vi "equipment_2.vi"() -> ()   [LabVIEW 2016]
uses:
  <vilib>/Platform/TimedLoop/XDataNode/timing_clust.ctl
  <vilib>/Platform/TimedLoop/XDataNode/nitl_modes.ctl
  <vilib>/Platform/TimedLoop/XDataNode/wakeup.ctl
  <instrlib>/Lake Shore 425/Public/Data/Field Data (Single Reading).vi
  <vilib>/platform/TimedLoop/XDataNode/XDataNode.xnode
  <instrlib>/Lake Shore 425/Lake Shore 425.lvlib
  <vilib>/Platform/TimedLoop/XDataNode/XDNodeRunTimeDep.lvlib
panel:
  out "Array":T1(array[cluster])
  out "XY Graph":T1(graph)
  in  "Period (ms)":i64
  out "Error":errorcluster
  in  "stop":bool
  out "Waveform Chart":dbl(graph)
  out "error out 3":errorcluster
  out "error out 2":errorcluster
  out "error out 1":errorcluster
  out "Probe Sensitivity 3":dbl=0.001 format="%^.3e"
  out "Probe Serial Number 3":string
  out "Probe Type  3":u16(ring)=40 items=["High Sensitivity"=40, "High Stability"=41, "Ultra-High Sensitivity"=42, "User Programmable Cable / High Sensitivity Probe"=50, "User Programmable Cable / High Stability Probe"=51, "User Programmable Cable / Ultra-High Sensitivity Probe"=52]
  out "Probe Sensitivity 2":dbl=0.001 format="%^.3e"
  out "Probe Serial Number 2":string
  out "Probe Type  2":u16(ring)=40 items=["High Sensitivity"=40, "High Stability"=41, "Ultra-High Sensitivity"=42, "User Programmable Cable / High Sensitivity Probe"=50, "User Programmable Cable / High Stability Probe"=51, "User Programmable Cable / Ultra-High Sensitivity Probe"=52]
  out "Probe Sensitivity":dbl=0.001 format="%^.3e"
  out "Probe Serial Number":string
  out "Probe Type":u16(ring)=40 items=["High Sensitivity"=40, "High Stability"=41, "Ultra-High Sensitivity"=42, "User Programmable Cable / High Sensitivity Probe"=50, "User Programmable Cable / High Stability Probe"=51, "User Programmable Cable / Ultra-High Sensitivity Probe"=52]
  in  "VISA Gaussmeter 3":refnum<visa-resource-name>
  in  "VISA Gaussmeter 2":refnum<visa-resource-name>
  in  "VISA Gaussmeter 1":refnum<visa-resource-name>
  in  "Gaussmeter 3":bool
  in  "Gaussmeter 2":bool
  in  "Gaussmeter 1":bool
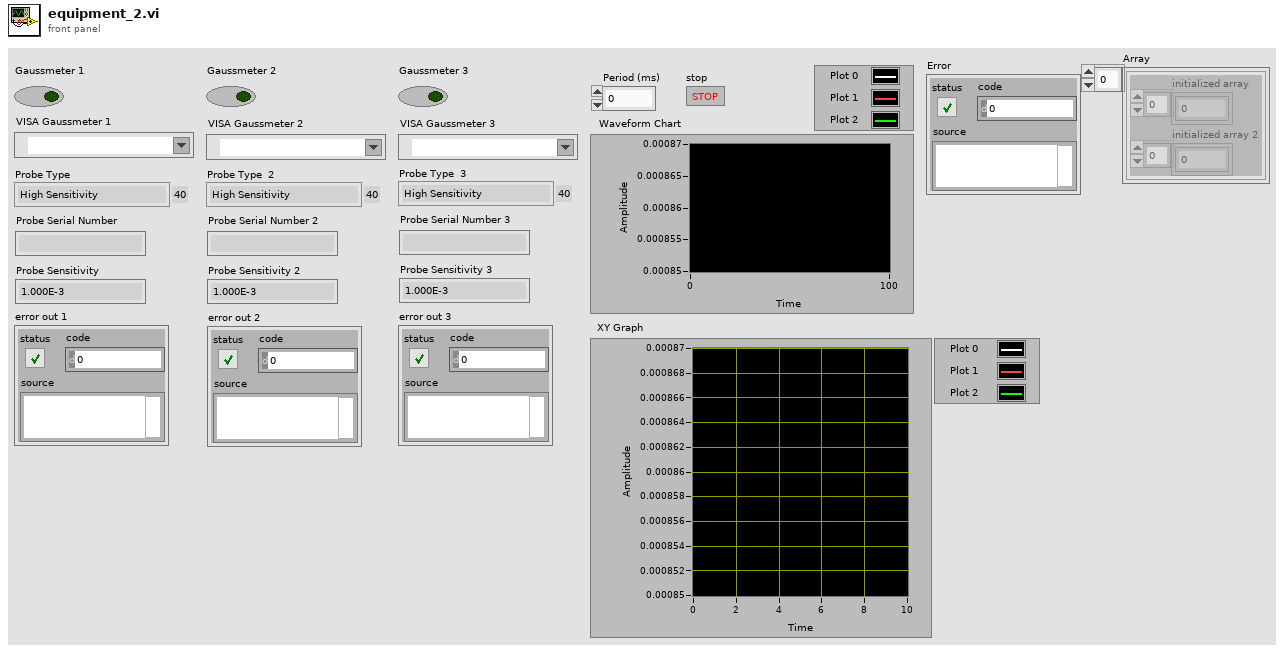
[diagram p1: front panel]
types:
  T1 = cluster{"initialized array":dbl[], "initialized array 2":dbl[]}[]
  T2 = typedef "XDNodeRunTimeDep.lvlib/timing_clust.ctl" = cluster{"Expected End [f-1]":u64, "Actual End [f-1]":u64, "Finished Late? [f-1]":bool, "Expected End [i-1]":u64, "Actual End [i-1]":u64, "Finished Late? [i-1]":bool, "Expected Start [i]":u64, "Actual Start [i]":u64, "Expected Start [f]":u64, "Actual Start [f]":u64, "Source Name":string, "Structure Name":string, "Period":i64, "Deadline":i64, "Offset":i64, "Start":i64, "Priority":i32, "Timeout":i32, "Mode":T3, "Wakeup Reason":T4, "Error":errorcluster, "Source Type":string, "Secondary Source Type":string, "Global End Time":u64, "Global Start Time":u64, "Frame Duration":u64, "Iteration Duration":u64, "Assigned CPU":i32, "I/O Scan Engine Mode":u32}
  T3 = typedef "XDNodeRunTimeDep.lvlib/nitl_modes.ctl" = enum32{"No Change", "Process missed periods, maintain original phase", "Discard missed periods, maintain original phase", "Process missed periods, ignore original phase", "Discard missed periods, ignore original phase"}
  T4 = typedef "XDNodeRunTimeDep.lvlib/wakeup.ctl" = enum32{"Normal", "Aborted", "Asynchronous wakeup", "Timing source error", "Timed loop error", "Timeout"}
  T5 = cluster{"initialized array":dbl[], "initialized array 2":dbl[]}
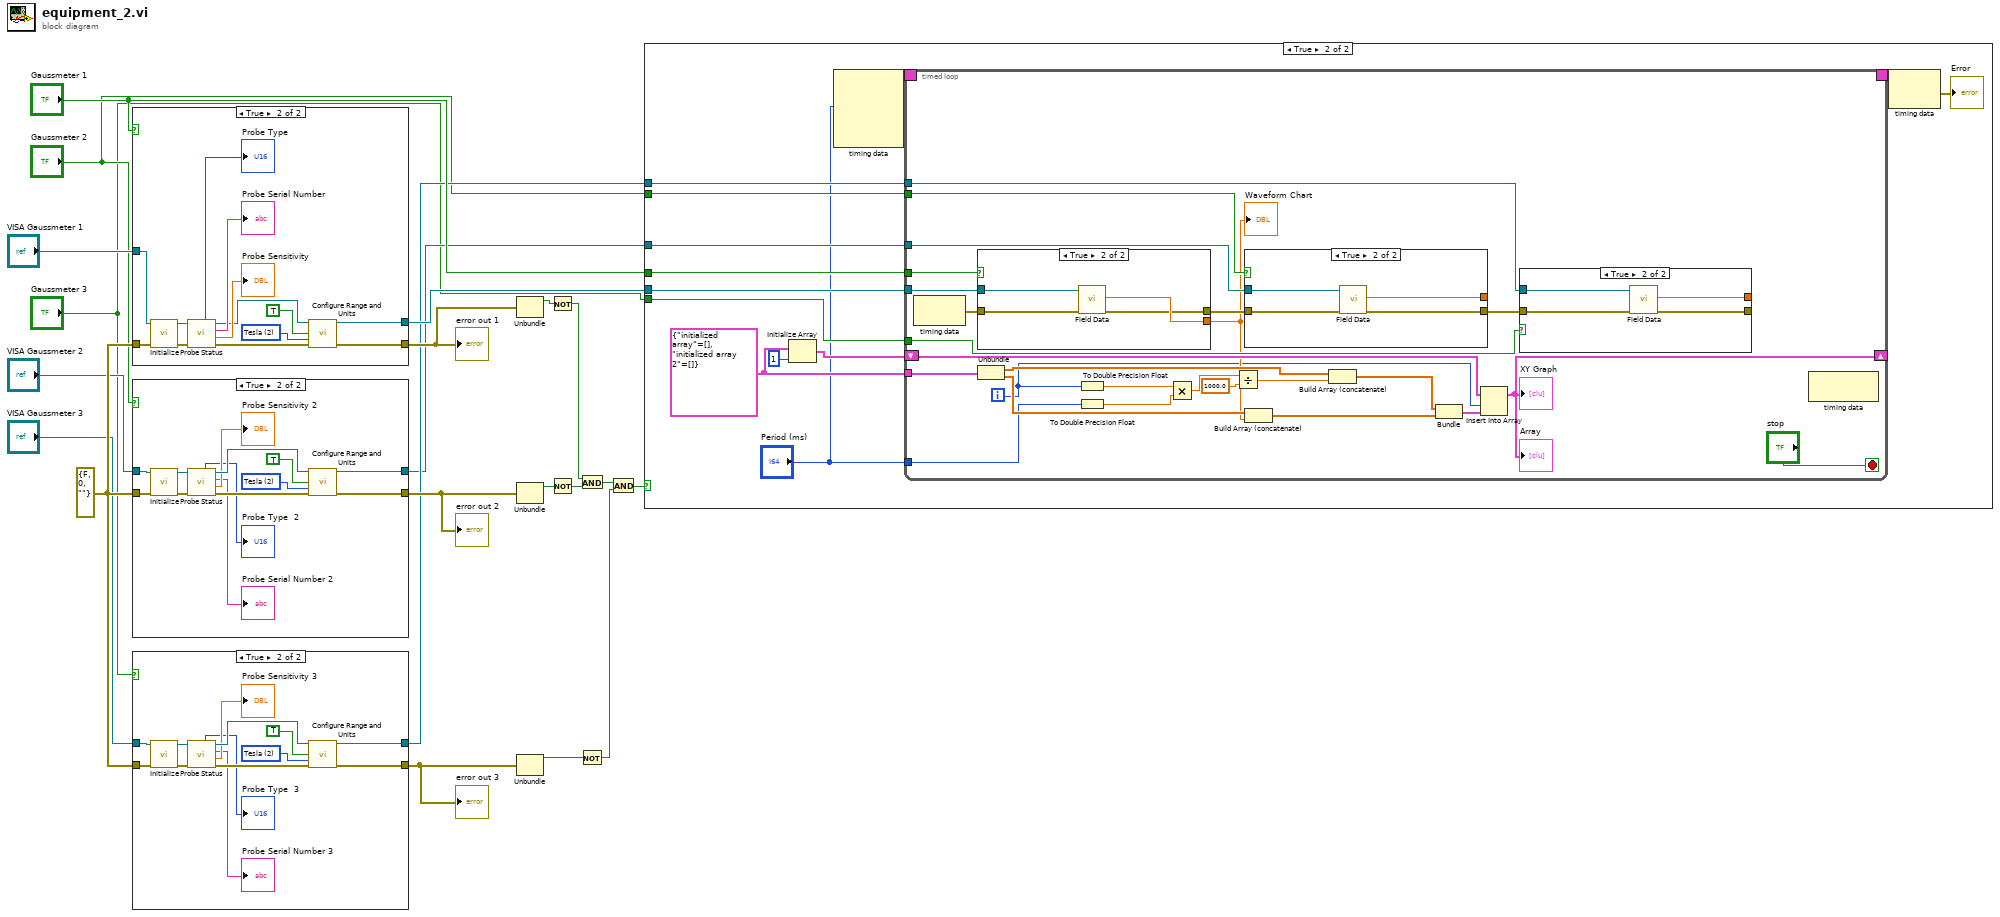
[diagram p0: block diagram]
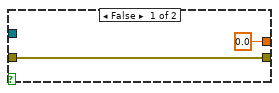
[diagram p3: hidden frame]
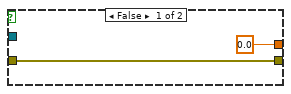
[diagram p4: hidden frame]
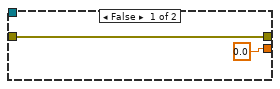
[diagram p5: hidden frame]
diagram:
  w21 = errorcluster {"status"=FALSE, "code"=0, "source"=""} ("error out")
  n1 = case shown="True" "Gaussmeter 1" {
    tunnel: [w23 w28] -> w15
    tunnel: w21 -> [w23 w36]
    tunnel: [w22 w25] -> w19
    tunnel: "VISA Gaussmeter 1" -> [w22 w24]
    frame False {
    }
    frame True {
      w26 = u16 2 items=["Gauss"=1, "Tesla"=2, "Oersted"=3, "Amp/meter"=4] ("Field Units (1:Gauss)")
      n2 = call <instrlib>:"Initialize.vi"("error in (no error)"=w36, "VISA resource name"=w24) -> ("error out"=w34:errorcluster, "VISA resource name out"=w35:refnum<visa-resource-name>)  [unwired: 8 in]
      n3 = call <instrlib>:"Probe Status.vi"("error in (no error)"=w34, "VISA resource name"=w35) -> ("error out"=w29:errorcluster, "Probe Sensitivity"=→"Probe Sensitivity":dbl, "Probe Serial Number"=→"Probe Serial Number":string, "VISA resource name out"=w30:refnum<visa-resource-name>, "Probe Type"=→"Probe Type":u16)  [unwired: 4 in, 1 out]
      n4 = call <instrlib>:"Configure Range and Units.vi"("VISA resource name"=w30, "Auto Range (F: Off)"=TRUE, "Field Units (1:Gauss)"=w26, "error in (no error)"=w29) -> ("VISA resource name out"=w25:refnum<visa-resource-name>, "error out"=w28:errorcluster)  [unwired: 10 in]
    }
  }
  "error out 1" <- w15
  n5 = case shown="True" "Gaussmeter 2" {
    tunnel: w21 -> [w38 w51]
    tunnel: [w38 w41] -> w14
    tunnel: "VISA Gaussmeter 2" -> [w37 w40]
    tunnel: [w37 w39] -> w3
    frame False {
    }
    frame True {
      w50 = u16 2 items=["Gauss"=1, "Tesla"=2, "Oersted"=3, "Amp/meter"=4] ("Field Units (1:Gauss)")
      n6 = call <instrlib>:"Initialize.vi"("error in (no error)"=w51, "VISA resource name"=w40) -> ("error out"=w42:errorcluster, "VISA resource name out"=w43:refnum<visa-resource-name>)  [unwired: 8 in]
      n7 = call <instrlib>:"Probe Status.vi"("error in (no error)"=w42, "VISA resource name"=w43) -> ("error out"=w48:errorcluster, "Probe Sensitivity"=→"Probe Sensitivity 2":dbl, "Probe Serial Number"=→"Probe Serial Number 2":string, "VISA resource name out"=w47:refnum<visa-resource-name>, "Probe Type"=→"Probe Type  2":u16)  [unwired: 4 in, 1 out]
      n8 = call <instrlib>:"Configure Range and Units.vi"("VISA resource name"=w47, "Auto Range (F: Off)"=TRUE, "Field Units (1:Gauss)"=w50, "error in (no error)"=w48) -> ("VISA resource name out"=w39:refnum<visa-resource-name>, "error out"=w41:errorcluster)  [unwired: 10 in]
    }
  }
  "error out 2" <- w14
  n9 = case shown="True" "Gaussmeter 3" {
    tunnel: w21 -> [w53 w66]
    tunnel: [w53 w58] -> w13
    tunnel: "VISA Gaussmeter 3" -> [w52 w55]
    tunnel: [w52 w54] -> w4
    frame False {
    }
    frame True {
      w65 = u16 2 items=["Gauss"=1, "Tesla"=2, "Oersted"=3, "Amp/meter"=4] ("Field Units (1:Gauss)")
      n10 = call <instrlib>:"Initialize.vi"("error in (no error)"=w66, "VISA resource name"=w55) -> ("error out"=w57:errorcluster, "VISA resource name out"=w56:refnum<visa-resource-name>)  [unwired: 8 in]
      n11 = call <instrlib>:"Probe Status.vi"("error in (no error)"=w57, "VISA resource name"=w56) -> ("error out"=w63:errorcluster, "Probe Sensitivity"=→"Probe Sensitivity 3":dbl, "Probe Serial Number"=→"Probe Serial Number 3":string, "VISA resource name out"=w62:refnum<visa-resource-name>, "Probe Type"=→"Probe Type  3":u16)  [unwired: 4 in, 1 out]
      n12 = call <instrlib>:"Configure Range and Units.vi"("VISA resource name"=w62, "Auto Range (F: Off)"=TRUE, "Field Units (1:Gauss)"=w65, "error in (no error)"=w63) -> ("VISA resource name out"=w54:refnum<visa-resource-name>, "error out"=w58:errorcluster)  [unwired: 10 in]
    }
  }
  "error out 3" <- w13
  n13 = Unbundle(w15) -> ("status"=w10:bool)  [unwired: 2 out]
  n14 = Unbundle(w14) -> ("status"=w8:bool)  [unwired: 2 out]
  n15 = Unbundle(w13) -> ("status"=w6:bool)  [unwired: 2 out]
  n16 = Not(x=w10) -> (.not. x?=w9:bool)
  n17 = Not(x=w8) -> (.not. x?=w7:bool)
  n18 = Not(x=w6) -> (.not. x?=w5:bool)
  n19 = And(x=w9, y=w7) -> (x .and. y?=w12:bool)
  n20 = And(x=w12, y=w5) -> (x .and. y?=w11:bool)
  n21 = case shown="True" w11 {
    tunnel: "Gaussmeter 1" -> [_ w77]
    tunnel: w19 -> [_ w75]
    tunnel: w4 -> [_ w73]
    tunnel: w3 -> [_ w74]
    tunnel: "Gaussmeter 2" -> [_ w72]
    tunnel: "Gaussmeter 3" -> [_ w71]
    frame False {
    }
    frame True {
      w68 = T5 {"initialized array"=[], "initialized array 2"=[]}
      n22 = Initialize Array(w68, 1) -> (w69:T1)
      n23 = node-c288("Period (ms)") -> (w79:T2)  [unwired: 3 in]
      n24 = timed-loop {
        timing: w79 -> [_]
        timing-out: [_] -> w78
        tunnel: w77 -> [w105]
        tunnel: w75 -> [w103]
        tunnel: w74 -> [w101]
        tunnel: w73 -> [w100]
        tunnel: w72 -> [w97]
        tunnel: w71 -> [w96]
        tunnel: w68 -> [w94]
        shift-right: [w88] -> _
        shift-left: w69 -> [w95]
        tunnel: "Period (ms)" -> [w83]
        i -> [w86]
        stop <- "stop" stop-if-true
        n25 = node-c288() -> (w102:errorcluster)  [unwired: 1 in]
        n26 = case shown="True" w105 {
          tunnel: w103 -> [_ w123]
          tunnel: [w119 w120] -> w99
          tunnel: w102 -> [w119 w122]
          tunnel: [0.0 ("Field Reading") w121] -> w87
          frame False {
          }
          frame True {
            n27 = call-poly <instrlib>:"Field Data.vi"("error in (no error)"=w122, "VISA resource name"=w123) -> ("error out"=w120:errorcluster, "Field Reading"=w121:dbl)  [unwired: 7 in, 1 out]
          }
        }
        "Waveform Chart" <- w87
        n28 = Unbundle(w94) -> ("initialized array"=w93:dbl[], "initialized array 2"=w92:dbl[])
        n29 = To Double Precision Float(number=w86) -> (double precision float=w85:dbl)
        n30 = To Double Precision Float(number=w83) -> (double precision float=w84:dbl)
        n31 = Multiply(x=w85, y=w84) -> (x*y=w82:dbl)
        n32 = Divide(x=w82, y=1000.0) -> (x/y=w81:dbl)
        n33 = case shown="True" w97 {
          tunnel: w101 -> [_ w117]
          tunnel: [w113 w116] -> w98
          tunnel: w99 -> [w113 w115]
          tunnel: [0.0 ("Field Reading") w114] -> _
          frame False {
          }
          frame True {
            n34 = call-poly <instrlib>:"Field Data.vi"("error in (no error)"=w115, "VISA resource name"=w117) -> ("error out"=w116:errorcluster, "Field Reading"=w114:dbl)  [unwired: 7 in, 1 out]
          }
        }
        n35 = Build Array (concatenate)(w92, w87) -> (w90:dbl[])
        n36 = Build Array (concatenate)(w93, w81) -> (w91:dbl[])
        n37 = Bundle(w91, w90) -> (w89:cluster{dbl[], dbl[]})  [unwired: 1 in]
        n38 = Insert Into Array(array=w95, index=w86, new element=w89) -> (w88:T1)
        "XY Graph" <- w88
        "Array" <- w88
        n39 = case shown="True" w96 {
          tunnel: w100 -> [_ w111]
          tunnel: [w107 w108] -> _
          tunnel: w98 -> [w107 w110]
          tunnel: [0.0 ("Field Reading") w109] -> _
          frame False {
          }
          frame True {
            n40 = call-poly <instrlib>:"Field Data.vi"("error in (no error)"=w110, "VISA resource name"=w111) -> ("error out"=w108:errorcluster, "Field Reading"=w109:dbl)  [unwired: 7 in, 1 out]
          }
        }
        n41 = node-c288() -> ()  [unwired: 1 in, 1 out]
      }
      n42 = node-c288(w78) -> (→"Error":errorcluster)
    }
  }
